vi "RSZVB Set Default Configuration State.vi"(8 "error in (no error)":errorcluster {"code" format="%.0x"}, 10 "Default Settings (T: On)":bool=TRUE, 11 "VISA session":refnum<visa-resource-name>) -> (0 "error out":errorcluster {"code" format="%.0x"}, 3 "dup VISA session":refnum<visa-resource-name>)   [LabVIEW 2011]
doc: "This VI overwrites the current settings of the multiport test set with the settings stored in the configuration file matrix.mtx. The file is stored in the directory C:\\Program Files\\Rohde&Schwarz\\Network Analyzer\\resources\\extdev. \n\nRemote-control command(s):\nROUTe<Ch>:CFILe ON | OFF"
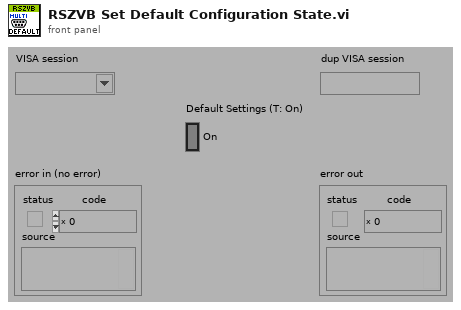
[diagram p1: front panel]
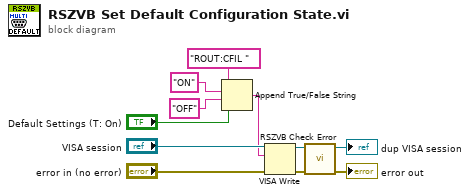
[diagram p0: block diagram]
diagram:
  n1 = Append True/False String(1:"Default Settings (T: On)", 2:"OFF" ("false string"), 3:"ON" ("true string"), 4:"ROUT:CFIL ") -> (0:w5:string)
  n2 = VISA Write(VISA resource name="VISA session", write buffer=w5, error in (no error)="error in (no error)") -> (VISA resource name out=w4:refnum<visa-resource-name>, error out=w3:errorcluster)  [unwired: 1 out]
  n3 = call "RSZVB Check Error.vi"("error in (no error)"=w3, "VISA session"=w4) -> ("error out"=→"error out":errorcluster, "dup VISA session"=→"dup VISA session":refnum<visa-resource-name>)  [unwired: 8 in]
